vi "List VIs without Test Coverage.vi"(8 "error in (no error)":errorcluster, 9 "Tests Root":path, 10 "Source Root":path) -> (0 "error out":errorcluster, 1 "Test VIs":path[](array[path]), 2 "VIs without test coverage":string[](array[string]))   [LabVIEW 2020]
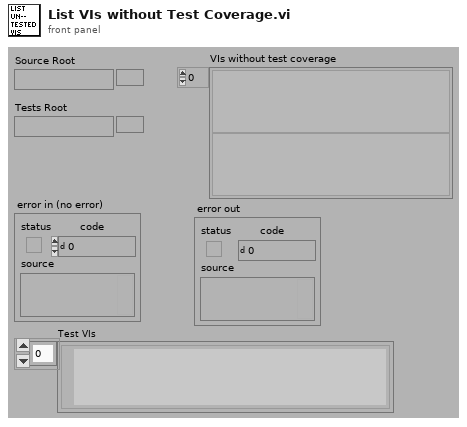
[diagram p1: front panel]
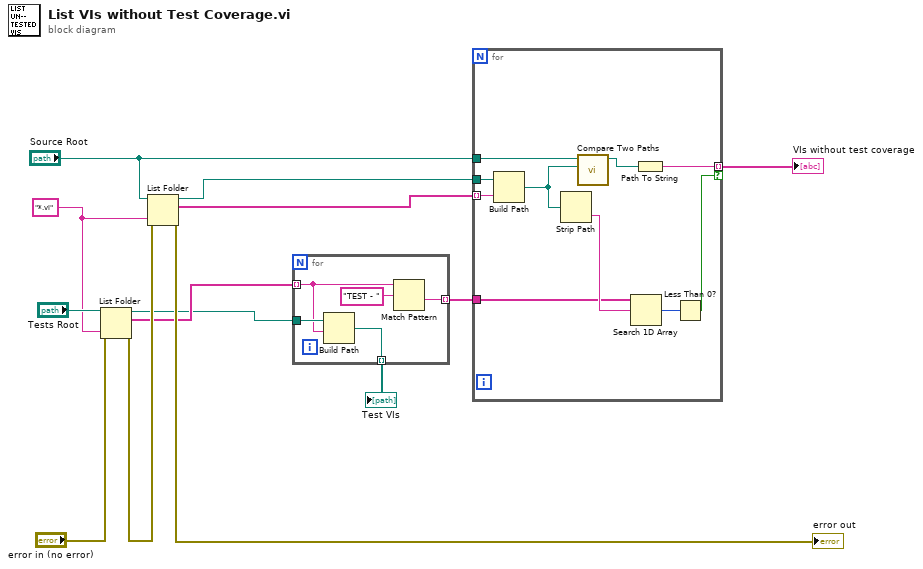
[diagram p0: block diagram]
diagram:
  w8 = "*.vi" ("pattern")
  n1 = List Folder(path="Tests Root", pattern=w8, error in="error in (no error)") -> (path out=w2:path, filenames=w5:string[], error out=w9:errorcluster)  [unwired: 1 in, 1 out]
  n2 = List Folder(path="Source Root", pattern=w8, error in=w9) -> (path out=w4:path, filenames=w3:string[], error out=→"error out":errorcluster)  [unwired: 1 in, 1 out]
  n3 = for {
    tunnel: w5 -> [w15] mode=indexing
    tunnel: [w17] -> w7 mode=indexing
    tunnel: w2 -> [w16]
    tunnel: [w14] -> w1 mode=indexing
    n4 = Build Path(base path=w16, name or relative path=w15) -> (appended path=w14:path)
    n5 = Match Pattern(string=w15, regular expression="TEST - ") -> (after substring=w17:string)  [unwired: 1 in, 3 out]
  }
  "Test VIs" <- w1
  n6 = for {
    tunnel: w7 -> [w27]
    tunnel: "Source Root" -> [w21]
    tunnel: [w25] -> w13 mode=indexing if=w22
    tunnel: w4 -> [w24]
    tunnel: w3 -> [w23] mode=indexing
    n7 = Build Path(base path=w24, name or relative path=w23) -> (appended path=w20:path)
    n8 = Strip Path(path=w20) -> (name=w28:string)  [unwired: 1 out]
    n9 = call <vilib>:"Compare Two Paths.vi"("Path 2"=w20, "Path 1"=w21) -> ("Relative Path from 1 to 2"=w19:path)  [unwired: 6 in, 3 out]
    n10 = Search 1D Array(1D array=w27, element=w28) -> (index of element=w26:i32)  [unwired: 1 in]
    n11 = Path To String(path=w19) -> (string=w25:string)
    n12 = Less Than 0?(x=w26) -> (x < 0?=w22:bool)
  }
  "VIs without test coverage" <- w13
